vi "log analysis_gps.vi"() -> ()   [LabVIEW 2018] (continued)
INS_RTKFIXED,37.37124990486,126.72244436292,7.9283,22.3000,-0.0470,0.2912,0.0231,-0.374405811,0.178417245,91.756627389,0.4699,0.2842,0.5361,0.1187,0.0913,0.0769,0.1664,0.1677,5.1090,0f000001,0*1daf5624\n\t", "INSPVAXA,USB3,0,47.5,FINESTEERING,2107,281654.050,02000000,471d,15824;INS_ALIGNMENT_COMPLETE,INS_RTKFIXED,37.37124978665,126.72244599017,7.9303,22.3000,-0.0443,0.2911,0.0221,-0.533917833,0.012272263,91.868776619,0.4905,0.2861,0.5500,0.1206,0.0913,0.0777,0.1663,0.1679,5.1083,0f000001,0*b5797700\n\t", "INSPVAXA,USB3,0,50.0,FINESTEERING,2107,281654.550,02000000,471d,15824;INS_ALIGNMENT_COMPLETE,INS_RTKFIXED,37.37124968143,126.72244761542,7.9319,22.3000,-0.0412,0.3115,0.0211,-0.670904223,-0.153080533,91.963880825,0.4905,0.2861,0.5500,0.1206,0.0913,0.0777,0.1663,0.1679,5.1083,0f000001,0*92b26d05\n\t", "INSPVAXA,USB3,0,50.0,FINESTEERING,2107,281655.050,02000000,471d,15824;INS_ALIGNMENT_COMPLETE,INS_RTKFIXED,37.37124956365,126.72244929570,7.9335,22.3000,-0.0287,0.2866,0.0163,-0.633101230,-0.384686660,92.084311938,0.4910,0.2854,0.5548,0.1194,0.0909,0.0776,0.1663,0.1676,5.1075,0f000001,0*34863e77\n\t", "INSPVAXA,USB3,0,45.0,FINESTEERING,2107,281655.550,02000000,471d,15824;INS_ALIGNMENT_COMPLETE,INS_RTKFIXED,37.37124945994,126.72245094764,7.9362,22.3000,-0.0311,0.2897,0.0132,-0.611375277,-0.501090520,92.141784733,0.4910,0.2854,0.5548,0.1194,0.0909,0.0776,0.1663,0.1676,5.1075,0f000001,0*d10d29d1\n\t", "INSPVAXA,USB3,0,45.0,FINESTEERING,2107,281656.050,02000000,471d,15824;INS_ALIGNMENT_COMPLETE,INS_RTKFIXED,37.37124935153,126.72245256975,7.9391,22.3000,-0.0386,0.2989,0.0132,-0.570389168,-0.459677112,92.213933334,0.4880,0.2845,0.5571,0.1182,0.0907,0.0775,0.1662,0.1674,5.1068,0f000001,0*a2bfb50c\n\t", "INSPVAXA,USB3,0,48.5,FINESTEERING,2107,281657.050,02000000,471d,15824;INS_ALIGNMENT_COMPLETE,INS_RTKFIXED,37.37124909812,126.72245582569,7.9380,22.3000,-0.0275,0.2897,0.0035,-0.469663173,-0.125718508,92.311505672,0.4756,0.2829,0.5533,0.1158,0.0905,0.0770,0.1661,0.1672,5.1057,0f000001,0*07acf302\n\t", "INSPVAXA,USB3,0,45.5,FINESTEERING,2107,281657.550,02000000,471d,15824;INS_ALIGNMENT_COMPLETE,INS_RTKFIXED,37.37124898406,126.72245743531,7.9384,22.3000,-0.0303,0.2838,-0.0006,-0.590912103,0.021707043,92.352601821,0.4756,0.2829,0.5533,0.1158,0.0905,0.0770,0.1661,0.1672,5.1057,0f000001,0*08773687\n\t", "INSPVAXA,USB3,0,45.5,FINESTEERING,2107,281658.050,02000000,471d,15824;INS_ALIGNMENT_COMPLETE,INS_RTKFIXED,37.37124887128,126.72245908204,7.9396,22.3000,-0.0216,0.3115,-0.0012,-0.683943291,-0.073848905,92.385513763,0.4705,0.2822,0.5519,0.1155,0.0906,0.0768,0.1661,0.1672,5.1055,0f000001,0*f6b19920\n\t", "INSPVAXA,USB3,0,47.0,FINESTEERING,2107,281658.550,02000000,471d,15824;INS_ALIGNMENT_COMPLETE,INS_RTKFIXED,37.37124877139,126.72246069396,7.9391,22.3000,-0.0206,0.3045,-0.0060,-0.740293612,-0.175653816,92.281973521,0.4705,0.2822,0.5519,0.1155,0.0906,0.0768,0.1661,0.1672,5.1055,0f000001,0*bcff9c67\n\t", "INSPVAXA,USB3,0,47.0,FINESTEERING,2107,281659.050,02000000,471d,15824;INS_ALIGNMENT_COMPLETE,INS_RTKFIXED,37.37124867854,126.72246232189,7.9387,22.3000,-0.0180,0.2907,0.0091,-0.761412694,-0.318240084,92.179006494,0.4753,0.2827,0.5554,0.1164,0.0908,0.0769,0.1661,0.1674,5.1056,0f000001,0*0b8ce59e\n\t", "INSPVAXA,USB3,0,48.0,FINESTEERING,2107,281660.050,02000000,471d,15824;INS_ALIGNMENT_COMPLETE,INS_RTKFIXED,37.37124847032,126.72246556404,7.9397,22.3000,-0.0209,0.3095,-0.0013,-0.677978130,-0.485395170,91.982371596,0.4840,0.2835,0.5609,0.1180,0.0910,0.0772,0.1661,0.1676,5.1059,0f000001,0*3e0b93c3\n\t", "INSPVAXA,USB3,0,49.0,FINESTEERING,2107,281660.550,02000000,471d,15824;INS_ALIGNMENT_COMPLETE,INS_RTKFIXED,37.37124837512,126.72246716631,7.9375,22.3000,-0.0227,0.2996,0.0028,-0.584311559,-0.386112040,91.866898679,0.4840,0.2835,0.5609,0.1180,0.0910,0.0772,0.1661,0.1676,5.1059,0f000001,0*45e2577e\n\t", "INSPVAXA,USB3,0,48.0,FINESTEERING,2107,281661.050,02000000,471d,15824;INS_ALIGNMENT_COMPLETE,INS_RTKFIXED,37.37124829104,126.72246876695,7.9348,22.3000,-0.0195,0.3013,0.0019,-0.605545922,-0.315098575,91.766604977,0.4893,0.2839,0.5649,0.1187,0.0910,0.0774,0.1661,0.1677,5.1061,0f000001,0*33d9cb01\n\t", "INSPVAXA,USB3,0,48.0,FINESTEERING,2107,281662.050,02000000,471d,15824;INS_ALIGNMENT_COMPLETE,INS_RTKFIXED,37.37124811177,126.72247195093,7.9364,22.3000,-0.0115,0.2979,0.0095,-0.572003488,-0.073343292,91.548333593,0.4907,0.2839,0.5665,0.1189,0.0910,0.0775,0.1660,0.1678,5.1065,0f000001,0*28865f95\n\t", "INSPVAXA,USB3,0,49.5,FINESTEERING,2107,281662.550,02000000,471d,15824;INS_ALIGNMENT_COMPLETE,INS_RTKFIXED,37.37124803275,126.72247354020,7.9355,22.3000,-0.0061,0.2831,0.0061,-0.496782272,0.001131440,91.456585867,0.4907,0.2839,0.5665,0.1189,0.0910,0.0775,0.1660,0.1678,5.1065,0f000001,0*47f56ed7\n\t", "INSPVAXA,USB3,0,49.5,FINESTEERING,2107,281663.050,02000000,471d,15824;INS_ALIGNMENT_COMPLETE,INS_RTKFIXED,37.37124795721,126.72247514952,7.9341,22.3000,-0.0032,0.2852,0.0045,-0.477077211,-0.102180757,91.467919397,0.4905,0.2838,0.5669,0.1189,0.0910,0.0775,0.1660,0.1678,5.1072,0f000001,0*7002819d\n\t", "INSPVAXA,USB3,0,50.0,FINESTEERING,2107,281663.550,02000000,471d,15824;INS_ALIGNMENT_COMPLETE,INS_RTKFIXED,37.37124785760,126.72247673495,7.9334,22.3000,-0.0075,0.2892,0.0034,-0.450270802,-0.044143313,91.482502163,0.4905,0.2838,0.5669,0.1189,0.0910,0.0775,0.1660,0.1678,5.1072,0f000001,0*8c44abc3\n\t", "INSPVAXA,USB3,0,49.0,FINESTEERING,2107,281666.550,02000000,471d,15824;INS_ALIGNMENT_COMPLETE,INS_RTKFIXED,37.37124721121,126.72248621902,7.9287,22.3000,-0.0121,0.2777,0.0145,-0.831221770,-0.084392330,92.040205552,0.4814,0.2826,0.5616,0.1182,0.0910,0.0772,0.1659,0.1677,5.1107,0f000001,0*a6e58744\n\t", "INSPVAXA,USB3,0,48.0,FINESTEERING,2107,281667.050,02000000,471d,15824;INS_ALIGNMENT_COMPLETE,INS_RTKFIXED,37.37124708689,126.72248776343,7.9278,22.3000,-0.0198,0.2843,0.0107,-0.784855196,-0.012804695,92.146893043,0.4774,0.2821,0.5586,0.1180,0.0910,0.0771,0.1659,0.1677,5.1116,0f000001,0*9d84455b\n\t", "INSPVAXA,USB3,0,47.0,FINESTEERING,2107,281669.550,02008000,471d,15824;INS_ALIGNMENT_COMPLETE,INS_RTKFIXED,37.37124639381,126.72249565319,7.9242,22.3000,-0.0324,0.2710,-0.0043,-0.728518677,-0.210964710,92.694614055,0.4668,0.2811,0.5506,0.1171,0.0909,0.0768,0.1658,0.1676,5.1128,0f000001,0*35942a2d\n\t", "INSPVAXA,USB3,0,45.0,FINESTEERING,2107,281671.050,02008000,471d,15824;INS_ALIGNMENT_COMPLETE,INS_RTKFIXED,37.37124595365,126.72250039060,7.9180,22.3000,-0.0288,0.2756,-0.0016,-0.760823395,-0.249987892,93.080464082,0.4568,0.2803,0.5426,0.1164,0.0907,0.0766,0.1658,0.1675,5.1134,0f000001,0*bc516aa8\n\t", "INSPVAXA,USB3,0,48.5,FINESTEERING,2107,281688.600,02000000,471d,15824;INS_ALIGNMENT_COMPLETE,INS_RTKFIXED,37.37124079033,126.72255707314,7.9955,22.3000,-0.0400,0.2827,0.0199,-0.588574844,-0.376557071,93.100954007,0.4119,0.2777,0.5056,0.1103,0.0901,0.0751,0.1654,0.1662,5.1286,0f000001,0*54052947\n\t", "INSPVAXA,USB3,0,49.0,FINESTEERING,2107,281692.600,02000000,471d,15824;INS_ALIGNMENT_COMPLETE,INS_RTKFIXED,37.37123920503,126.72256999557,8.0063,22.3000,-0.0578,0.2919,0.0133,-0.505898312,-0.718535643,95.167243727,0.4145,0.2869,0.5143,0.1104,0.0917,0.0756,0.1655,0.1660,5.1296,0f000001,0*c2aa46e2\n\t", "INSPVAXA,USB3,0,47.0,FINESTEERING,2107,281695.100,02000000,471d,15824;INS_ALIGNMENT_COMPLETE,INS_RTKFIXED,37.37123802053,126.72257797318,8.0018,22.3000,-0.0593,0.2857,0.0050,-0.558480992,-0.544515597,95.936874114,0.4188,0.2924,0.5242,0.1107,0.0922,0.0760,0.1653,0.1660,5.1321,0f000001,0*63dd8461\n\t", "INSPVAXA,USB3,0,50.0,FINESTEERING,2107,281696.100,02000000,471d,15824;INS_ALIGNMENT_COMPLETE,INS_RTKFIXED,37.37123750613,126.72258125435,8.0103,22.3000,-0.0675,0.2976,0.0099,-0.630143652,-0.426020851,96.136843189,0.4217,0.2975,0.5312,0.1110,0.0928,0.0763,0.1653,0.1661,5.1333,0f000001,0*1735351b\n\t", "INSPVAXA,USB3,0,48.0,FINESTEERING,2107,281697.100,02000000,471d,15824;INS_ALIGNMENT_COMPLETE,INS_RTKFIXED,37.37123698193,126.72258460282,8.0164,22.3000,-0.0758,0.2921,0.0167,-0.785011326,-0.362402901,96.082518685,0.4231,0.3001,0.5368,0.1110,0.0930,0.0765,0.1653,0.1661,5.1347,0f000001,0*98f592bb\n\t", "INSPVAXA,USB3,0,46.0,FINESTEERING,2107,281698.600,02000000,471d,15824;INS_ALIGNMENT_COMPLETE,INS_RTKFIXED,37.37123629785,126.72258936520,8.0229,22.3000,-0.0531,0.2999,0.0083,-0.429170205,-0.373001381,94.965510664,0.4234,0.2998,0.5394,0.1109,0.0928,0.0765,0.1652,0.1661,5.1363,0f000001,0*f47145af\n\t", "INSPVAXA,USB3,0,47.5,FINESTEERING,2107,281699.100,02000000,471d,15824;INS_ALIGNMENT_COMPLETE,INS_RTKFIXED,37.37123609876,126.72259093053,8.0227,22.3000,-0.0510,0.2765,0.0255,-0.446439369,-0.329194520,94.348853221,0.4489,0.3061,0.5623,0.1153,0.0940,0.0781,0.1653,0.1666,5.1379,0f000001,0*f0667120\n\t", "INSPVAXA,USB3,0,47.5,FINESTEERING,2107,281699.600,02000000,471d,15824;INS_ALIGNMENT_COMPLETE,INS_RTKFIXED,37.37123591668,126.72259250997,8.0220,22.3000,-0.0473,0.2889,0.0139,-0.571559626,-0.354554479,93.825556987,0.4489,0.3061,0.5623,0.1153,0.0940,0.0781,0.1653,0.1666,5.1379,0f000001,0*d2b474b3\n\t", "INSPVAXA,USB3,0,46.5,FINESTEERING,2107,281701.100,02000000,471d,15824;INS_ALIGNMENT_COMPLETE,INS_RTKFIXED,37.37123543674,126.72259726700,8.0121,22.3000,-0.0545,0.2706,0.0002,-0.599049195,-0.261744490,92.339458537,0.4977,0.3169,0.6162,0.1213,0.0953,0.0812,0.1655,0.1673,5.1411,0f000001,0*bffa09db\n\t", "INSPVAXA,USB3,0,46.5,FINESTEERING,2107,281701.600,02000000,471d,15824;INS_ALIGNMENT_COMPLETE,INS_RTKFIXED,37.37123527924,126.72259888049,8.0099,22.3000,-0.0672,0.2799,0.0012,-0.451214464,-0.240273754,91.937158376,0.4977,0.3169,0.6162,0.1213,0.0953,0.0812,0.1655,0.1673,5.1411,0f000001,0*07d7c6e7\n\t", "INSPVAXA,USB3,0,47.5,FINESTEERING,2107,281702.100,02000000,471d,15824;INS_ALIGNMENT_COMPLETE,INS_RTKFIXED,37.37123511620,126.72260050182,8.0076,22.3000,-0.0639,0.2800,0.0071,-0.195522404,-0.345413269,91.687324212,0.5177,0.3188,0.6402,0.1229,0.0952,0.0822,0.1654,0.1675,5.1426,0f000001,0*c86b297b\n\t", "INSPVAXA,USB3,0,47.5,FINESTEERING,2107,281702.600,02000000,471d,15824;INS_ALIGNMENT_COMPLETE,INS_RTKFIXED,37.37123499980,126.72260210723,8.0027,22.3000,-0.0718,0.2769,0.0046,-0.302041493,-0.225202254,91.651416522,0.5177,0.3188,0.6402,0.1229,0.0952,0.0822,0.1654,0.1675,5.1426,0f000001,0*8e66a9f4\n\t", "INSPVAXA,USB3,0,45.0,FINESTEERING,2107,281703.100,02000000,471d,15824;INS_ALIGNMENT_COMPLETE,INS_RTKFIXED,37.37123487466,126.72260370060,7.9985,22.3000,-0.0709,0.2986,0.0115,-0.451708680,-0.253518479,91.680936337,0.5338,0.3195,0.6613,0.1238,0.0951,0.0829,0.1654,0.1676,5.1442,0f000001,0*4cdf9694\n\t", "INSPVAXA,USB3,0,45.0,FINESTEERING,2107,281703.600,02000000,471d,15824;INS_ALIGNMENT_COMPLETE,INS_RTKFIXED,37.37123473881,126.72260531876,7.9953,22.3000,-0.0686,0.2839,0.0069,-0.545599376,-0.327030847,91.675911567,0.5338,0.3195,0.6613,0.1238,0.0951,0.0829,0.1654,0.1676,5.1442,0f000001,0*45031f18\n\t", "INSPVAXA,USB3,0,49.0,FINESTEERING,2107,281704.100,02000000,471d,15824;INS_ALIGNMENT_COMPLETE,INS_RTKFIXED,37.37123458474,126.72260693238,7.9920,22.3000,-0.0673,0.2665,0.0075,-0.425050811,-0.262256492,91.709435128,0.4707,0.3025,0.6068,0.1142,0.0929,0.0788,0.1651,0.1663,5.1457,0f000001,0*e320c835\n\t", "INSPVAXA,USB3,0,49.0,FINESTEERING,2107,281704.600,02000000,471d,15824;INS_ALIGNMENT_COMPLETE,INS_RTKFIXED,37.37123444909,126.72260850935,7.9897,22.3000,-0.0657,0.2780,0.0024,-0.316216564,-0.175738279,91.794051031,0.4707,0.3025,0.6068,0.1142,0.0929,0.0788,0.1651,0.1663,5.1457,0f000001,0*c024accc\n\t", "INSPVAXA,USB3,0,48.5,FINESTEERING,2107,281705.100,02000000,471d,15824;INS_ALIGNMENT_COMPLETE,INS_RTKFIXED,37.37123430154,126.72261008444,7.9873,22.3000,-0.0633,0.2873,0.0036,-0.217542977,-0.113568421,91.893535267,0.4436,0.2955,0.5802,0.1116,0.0926,0.0771,0.1650,0.1661,5.1471,0f000001,0*d440002a\n\t", "INSPVAXA,USB3,0,48.5,FINESTEERING,2107,281705.600,02000000,471d,15824;INS_ALIGNMENT_COMPLETE,INS_RTKFIXED,37.37123415162,126.72261168716,7.9829,22.3000,-0.0703,0.2649,-0.0005,-0.095589755,-0.218915380,92.040147564,0.4436,0.2955,0.5802,0.1116,0.0926,0.0771,0.1650,0.1661,5.1471,0f000001,0*3cc5b35f\n\t", "INSPVAXA,USB3,0,47.0,FINESTEERING,2107,281706.100,02000000,471d,15824;INS_ALIGNMENT_COMPLETE,INS_RTKFIXED,37.37123399063,126.72261326131,7.9791,22.3000,-0.0689,0.2735,0.0004,-0.068217682,-0.338302495,92.198825064,0.4298,0.2917,0.5629,0.1111,0.0926,0.0763,0.1650,0.1662,5.1486,0f000001,0*0d2ba2e9\n\t", "INSPVAXA,USB3,0,47.0,FINESTEERING,2107,281706.600,02000000,471d,15824;INS_ALIGNMENT_COMPLETE,INS_RTKFIXED,37.37123384411,126.72261483687,7.9751,22.3000,-0.0650,0.2968,0.0010,-0.179433418,-0.243858761,92.416884280,0.4298,0.2917,0.5629,0.1111,0.0926,0.0763,0.1650,0.1662,5.1486,0f000001,0*3a14ca69\n\t", "INSPVAXA,USB3,0,46.5,FINESTEERING,2107,281707.100,02000000,471d,15824;INS_ALIGNMENT_COMPLETE,INS_RTKFIXED,37.37123367618,126.72261651459,7.9700,22.3000,-0.0663,0.2892,-0.0095,-0.200364886,-0.287717605,92.565518940,0.4222,0.2895,0.5502,0.1114,0.0926,0.0759,0.1650,0.1662,5.1501,0f000001,0*7d04a348\n\t", "INSPVAXA,USB3,0,46.5,FINESTEERING,2107,281707.600,02000000,471d,15824;INS_ALIGNMENT_COMPLETE,INS_RTKFIXED,37.37123350681,126.72261819185,7.9654,22.3000,-0.0701,0.2829,0.0020,-0.131719254,-0.267188121,92.719108134,0.4222,0.2895,0.5502,0.1114,0.0926,0.0759,0.1650,0.1662,5.1501,0f000001,0*336f6954\n\t", "INSPVAXA,USB3,0,46.5,FINESTEERING,2107,281708.100,02008000,471d,15824;INS_ALIGNMENT_COMPLETE,INS_RTKFIXED,37.37123332387,126.72261975086,7.9614,22.3000,-0.0675,0.2853,0.0025,-0.071583190,-0.126032206,92.932636241,0.4187,0.2881,0.5409,0.1120,0.0926,0.0757,0.1650,0.1662,5.1517,0f000001,0*717a5375\n\t", "INSPVAXA,USB3,0,44.5,FINESTEERING,2107,281708.600,02008000,471d,15824;INS_ALIGNMENT_COMPLETE,INS_RTKFIXED,37.37123313227,126.72262135847,7.9570,22.3000,-0.0735,0.2879,0.0053,-0.006863606,-0.144876749,93.163596493,0.4187,0.2881,0.5409,0.1120,0.0926,0.0757,0.1650,0.1662,5.1517,0f000001,0*5328ad5b\n\t", "INSPVAXA,USB3,0,45.0,FINESTEERING,2107,281709.100,02008000,471d,15824;INS_ALIGNMENT_COMPLETE,INS_RTKFIXED,37.37123292904,126.72262301314,7.9519,22.3000,-0.0859,0.2798,0.0008,-0.080624798,-0.243890207,93.431588866,0.4168,0.2866,0.5328,0.1122,0.0923,0.0756,0.1650,0.1661,5.1533,0f000001,0*5e6ee30b\n\t", "INSPVAXA,USB3,0,45.0,FINESTEERING,2107,281709.600,02008000,471d,15824;INS_ALIGNMENT_COMPLETE,INS_RTKFIXED,37.37123275225,126.72262461471,7.9473,22.3000,-0.0829,0.2713,-0.0040,-0.149358912,-0.219762797,93.778103830,0.4168,0.2866,0.5328,0.1122,0.0923,0.0756,0.1650,0.1661,5.1533,0f000001,0*a588a807\n\t", "INSPVAXA,USB3,0,45.0,FINESTEERING,2107,281710.100,02008000,471d,15824;INS_ALIGNMENT_COMPLETE,INS_RTKFIXED,37.37123256909,126.72262620659,7.9441,22.3000,-0.0800,0.2841,-0.0050,-0.348638579,-0.216651585,94.159342839,0.4165,0.2852,0.5266,0.1124,0.0920,0.0756,0.1649,0.1660,5.1550,0f000001,0*bff3e08f\n\t", "INSPVAXA,USB3,0,49.0,FINESTEERING,2107,281710.600,02008000,471d,15824;INS_ALIGNMENT_COMPLETE,INS_RTKFIXED,37.37123239058,126.72262777304,7.9409,22.3000,-0.0798,0.2944,-0.0023,-0.430611394,-0.234860716,94.547061846,0.4165,0.2852,0.5266,0.1124,0.0920,0.0756,0.1649,0.1660,5.1550,0f000001,0*d6308b3b\n\t", "DUALANTENNAHEADINGA,USB3,0,48.0,FINESTEERING,2107,281711.100,02008000,d426,15824;SOL_COMPUTED,NARROW_FLOAT,-1.000000000,80.289344788,-44.356048584,0.0,300.718536377,180.000000000,\"631T\",19,8,8,8,04,00,20,23*d9de486e\n\t", "INSPVAXA,USB3,0,48.0,FINESTEERING,2107,281711.600,02008000,471d,15824;INS_ALIGNMENT_COMPLETE,INS_RTKFIXED,37.37123199532,126.72263088788,7.9365,22.3000,-0.0807,0.2590,-0.0074,-0.567150366,-0.272813348,95.297147623,0.4157,0.2838,0.5214,0.1122,0.0917,0.0756,0.1649,0.1659,5.1567,0f000001,0*5002614b\n\t", "INSPVAXA,USB3,0,47.5,FINESTEERING,2107,281712.100,02000000,471d,15824;INS_ALIGNMENT_COMPLETE,INS_RTKFIXED,37.37123179004,126.72263242494,7.9368,22.3000,-0.0695,0.2725,-0.0019,-0.650599321,-0.130078123,95.641509239,0.4157,0.2825,0.5179,0.1119,0.0914,0.0757,0.1648,0.1658,5.1583,0f000001,0*44de4a90\n\t", "INSPVAXA,USB3,0,47.5,FINESTEERING,2107,281712.600,02000000,471d,15824;INS_ALIGNMENT_COMPLETE,INS_RTKFIXED,37.37123168411,126.72263304090,7.9346,22.3000,-0.0497,-0.0387,-0.0006,-0.768033993,-0.261504929,95.591408924,0.4157,0.2825,0.5179,0.1119,0.0914,0.0757,0.1648,0.1658,5.1583,0f000001,0*fe46b876\n\t", "INSPVAXA,USB3,0,49.0,FINESTEERING,2107,281713.100,02000000,471d,15824;INS_ALIGNMENT_COMPLETE,INS_RTKFIXED,37.37123162730,126.72263286916,7.9326,22.3000,-0.0467,-0.0089,-0.0011,-0.752184115,-0.247755356,95.681640614,0.4152,0.2811,0.5147,0.1145,0.0912,0.0757,0.1647,0.1656,5.1599,0f000001,0*7f213a14\n\t", "INSPVAXA,USB3,0,49.0,FINESTEERING,2107,281713.600,02000000,471d,15824;INS_ALIGNMENT_COMPLETE,INS_RTKFIXED,37.37123160226,126.72263284212,7.9312,22.3000,-0.0436,-0.0236,-0.0010,-0.754995173,-0.249841362,95.676005261,0.4152,0.2811,0.5147,0.1145,0.0912,0.0757,0.1647,0.1656,5.1599,0f000001,0*48133efc\n\t", "INSPVAXA,USB3,0,49.0,FINESTEERING,2107,281714.100,02000000,471d,15824;INS_ALIGNMENT_COMPLETE,INS_RTKFIXED,37.37123158399,126.72263279406,7.9298,22.3000,-0.0399,-0.0233,-0.0008,-0.760010437,-0.248532428,95.678009350,0.4172,0.2798,0.5120,0.1137,0.0910,0.0756,0.1647,0.1655,5.1584,0f000001,0*814e0d11\n\t", "INSPVAXA,USB3,0,49.0,FINESTEERING,2107,281714.600,02000000,471d,15824;INS_ALIGNMENT_COMPLETE,INS_RTKFIXED,37.37123160799,126.72263276180,7.9284,22.3000,-0.0364,-0.0240,-0.0004,-0.762178806,-0.247643160,95.688059791,0.4172,0.2798,0.5120,0.1137,0.0910,0.0756,0.1647,0.1655,5.1584,0f000001,0*b1bc14cf\n\t", "INSPVAXA,USB3,0,47.5,FINESTEERING,2107,281715.100,02000000,471d,15824;INS_ALIGNMENT_COMPLETE,INS_RTKFIXED,37.37123162975,126.72263271812,7.9272,22.3000,-0.0332,-0.0254,0.0000,-0.763298909,-0.246600758,95.701763966,0.4185,0.2789,0.5100,0.1127,0.0908,0.0756,0.1646,0.1655,5.1528,0f000001,0*0879a17d\n\t", "INSPVAXA,USB3,0,47.5,FINESTEERING,2107,281715.600,02000000,471d,15824;INS_ALIGNMENT_COMPLETE,INS_RTKFIXED,37.37123166929,126.72263269074,7.9254,22.3000,-0.0295,-0.0259,0.0000,-0.763181363,-0.245447561,95.720594560,0.4185,0.2789,0.5100,0.1127,0.0908,0.0756,0.1646,0.1655,5.1528,0f000001,0*8b144437\n\t", "INSPVAXA,USB3,0,47.5,FINESTEERING,2107,281716.100,02000000,471d,15824;INS_ALIGNMENT_COMPLETE,INS_RTKFIXED,37.37123170967,126.72263265292,7.9238,22.3000,-0.0264,-0.0269,-0.0004,-0.764362400,-0.245981262,95.737150322,0.4185,0.2781,0.5083,0.1118,0.0906,0.0755,0.1646,0.1654,5.1445,0f000001,0*f8e3de3b\n\t", "INSPVAXA,USB3,0,48.5,FINESTEERING,2107,281716.600,02000000,471d,15824;INS_ALIGNMENT_COMPLETE,INS_RTKFIXED,37.37123176851,126.72263264285,7.9224,22.3000,-0.0232,-0.0258,0.0004,-0.768584569,-0.246689742,95.757168230,0.4185,0.2781,0.5083,0.1118,0.0906,0.0755,0.1646,0.1654,5.1445,0f000001,0*4a6b11ff\n\t", "INSPVAXA,USB3,0,45.5,FINESTEERING,2107,281717.100,02000000,471d,15824;INS_ALIGNMENT_COMPLETE,INS_RTKFIXED,37.37123177555,126.72263328033,7.9223,22.3000,-0.0576,0.3644,0.0001,-0.832005766,-0.123893266,96.001595857,0.4179,0.2777,0.5069,0.1104,0.0904,0.0755,0.1645,0.1655,5.1359,0f000001,0*38e87445\n\t", "INSPVAXA,USB3,0,45.5,FINESTEERING,2107,281717.600,02000000,471d,15824;INS_ALIGNMENT_COMPLETE,INS_RTKFIXED,37.37123167276,126.72263519972,7.9226,22.3000,-0.0392,0.2146,0.0043,-0.709863436,-0.109995299,96.136679690,0.4179,0.2777,0.5069,0.1104,0.0904,0.0755,0.1645,0.1655,5.1359,0f000001,0*131293dc\n\t", "INSPVAXA,USB3,0,50.0,FINESTEERING,2107,281718.100,02000000,471d,15824;INS_ALIGNMENT_COMPLETE,INS_RTKFIXED,37.37123162511,126.72263648434,7.9220,22.3000,-0.0555,0.3053,-0.0001,-0.719313500,0.029309323,96.356461624,0.4142,0.2776,0.5061,0.1102,0.0903,0.0754,0.1645,0.1655,5.1346,0f000001,0*65443b6e\n\t", "INSPVAXA,USB3,0,50.0,FINESTEERING,2107,281718.600,02000000,471d,15824;INS_ALIGNMENT_COMPLETE,INS_RTKFIXED,37.37123150821,126.72263819990,7.9208,22.3000,-0.0327,0.2368,0.0101,-0.836011591,-0.122473478,96.522319824,0.4142,0.2776,0.5061,0.1102,0.0903,0.0754,0.1645,0.1655,5.1346,0f000001,0*3c509359\n\t", "DUALANTENNAHEADINGA,USB3,0,50.0,FINESTEERING,2107,281719.100,02000000,d426,15824;SOL_COMPUTED,NARROW_FLOAT,-1.000000000,81.686454773,-57.139007568,0.0,241.198776245,172.427688599,\"631T\",19,9,9,9,04,00,20,23*98acc785\n\t", "DUALANTENNAHEADINGA,USB3,0,50.5,FINESTEERING,2107,281719.600,02000000,d426,15824;SOL_COMPUTED,NARROW_FLOAT,-1.000000000,81.772033691,-56.640899658,0.0,242.991180420,178.717849731,\"631T\",19,9,9,9,04,00,20,23*247738d5\n\t", "DUALANTENNAHEADINGA,USB3,0,50.5,FINESTEERING,2107,281720.100,02000000,d426,15824;SOL_COMPUTED,NARROW_FLOAT,-1.000000000,77.492141724,-53.828643799,0.0,241.831039429,180.000000000,\"631T\",18,8,8,8,04,00,20,23*d2631c09\n\t", "INSPVAXA,USB3,0,50.5,FINESTEERING,2107,281720.600,02000000,471d,15824;INS_ALIGNMENT_COMPLETE,INS_RTKFIXED,37.37123091097,126.72264464380,7.9199,22.3000,-0.0398,0.2663,0.0043,-0.781491920,-0.508123165,97.323827994,0.4101,0.2774,0.5047,0.1107,0.0902,0.0753,0.1644,0.1655,5.1368,0f000001,0*f5b81503\n\t", "INSPVAXA,USB3,0,44.0,FINESTEERING,2107,281721.100,02000000,471d,15824;INS_ALIGNMENT_COMPLETE,INS_RTKFIXED,37.37123072966,126.72264623422,7.9185,22.3000,-0.0371,0.2532,0.0002,-0.791450093,-0.646314917,97.497529339,0.4089,0.2773,0.5042,0.1108,0.0902,0.0752,0.1643,0.1654,5.1370,0f000001,0*861aa27e\n\t", "INSPVAXA,USB3,0,44.0,FINESTEERING,2107,281721.600,02000000,471d,15824;INS_ALIGNMENT_COMPLETE,INS_RTKFIXED,37.37123052324,126.72264786246,7.9181,22.3000,-0.0351,0.2700,-0.0076,-0.812155960,-0.930405893,97.703567688,0.4089,0.2773,0.5042,0.1108,0.0902,0.0752,0.1643,0.1654,5.1370,0f000001,0*0ebef3fd\n\t", "DUALANTENNAHEADINGA,USB3,0,44.0,FINESTEERING,2107,281722.100,02000000,d426,15824;SOL_COMPUTED,NARROW_FLOAT,-1.000000000,76.782913208,-57.608184814,0.0,174.641418457,168.358657837,\"631T\",20,9,9,9,04,00,20,23*2ea8cf0f\n\t", "INSPVAXA,USB3,0,47.5,FINESTEERING,2107,281722.600,02000000,471d,15824;INS_ALIGNMENT_COMPLETE,INS_RTKFIXED,37.37123005820,126.72265110077,7.9161,22.3000,-0.0311,0.2570,0.0035,-0.906537656,-1.041249846,98.071868373,0.4085,0.2773,0.5040,0.1115,0.0902,0.0751,0.1642,0.1654,5.1358,0f000001,0*21f04e37\n\t", "INSPVAXA,USB3,0,46.5,FINESTEERING,2107,281723.100,02000000,471d,15824;INS_ALIGNMENT_COMPLETE,INS_RTKFIXED,37.37122980766,126.72265265100,7.9163,22.3000,-0.0386,0.2513,-0.0019,-0.889198276,-0.870105161,98.274091102,0.4388,0.2808,0.5181,0.1159,0.0909,0.0762,0.1643,0.1660,5.1342,0f000001,0*96582036\n\t", "INSPVAXA,USB3,0,46.5,FINESTEERING,2107,281723.600,02000000,471d,15824;INS_ALIGNMENT_COMPLETE,INS_RTKFIXED,37.37122953819,126.72265422237,7.9162,22.3000,-0.0387,0.2553,0.0003,-0.677469280,-0.596133835,98.468377537,0.4388,0.2808,0.5181,0.1159,0.0909,0.0762,0.1643,0.1660,5.1342,0f000001,0*0344c34f\n\t", "INSPVAXA,USB3,0,50.0,FINESTEERING,2107,281724.100,02000000,471d,15824;INS_ALIGNMENT_COMPLETE,INS_RTKFIXED,37.37122926408,126.72265582006,7.9155,22.3000,-0.0392,0.2664,0.0052,-0.552231420,-0.356374368,98.612981561,0.4681,0.2838,0.5347,0.1192,0.0914,0.0772,0.1643,0.1664,5.1316,0f000001,0*5ab7c900\n\t", "DUALANTENNAHEADINGA,USB3,0,50.0,FINESTEERING,2107,281724.600,02000000,d426,15824;SOL_COMPUTED,NARROW_FLOAT,-1.000000000,73.725341797,-44.577819824,0.0,216.156219482,180.000000000,\"631T\",18,6,6,6,04,00,20,03*eb9ec7a2\n\t", "DUALANTENNAHEADINGA,USB3,0,48.0,FINESTEERING,2107,281725.100,02000000,d426,15824;SOL_COMPUTED,NARROW_FLOAT,-1.000000000,77.386466980,-38.596252441,0.0,347.977569580,180.000000000,\"631T\",17,7,7,6,04,00,20,33*9a5ac747\n\t", "DUALANTENNAHEADINGA,USB3,0,48.0,FINESTEERING,2107,281725.600,02000000,d426,15824;SOL_COMPUTED,NARROW_FLOAT,-1.000000000,74.226867676,-38.265563965,0.0,314.182830811,180.000000000,\"631T\",17,7,7,6,04,00,20,23*45cb672d\n\t", "DUALANTENNAHEADINGA,USB3,0,48.0,FINESTEERING,2107,281726.100,02000000,d426,15824;SOL_COMPUTED,NARROW_FLOAT,-1.000000000,204.498168945,55.872886658,0.0,207.629287720,89.946952820,\"631T\",18,5,5,5,04,00,20,03*b03bb7fc\n\t", "DUALANTENNAHEADINGA,USB3,0,49.5,FINESTEERING,2107,281726.600,02000000,d426,15824;SOL_COMPUTED,NARROW_FLOAT,-1.000000000,205.496963501,57.094558716,0.0,186.765380859,78.783508301,\"631T\",22,5,5,5,04,00,20,03*8aea4973\n\t", "INSPVAXA,USB3,0,40.0,FINESTEERING,2107,281727.100,02000000,471d,15824;INS_ALIGNMENT_COMPLETE,INS_RTKFIXED,37.37122812563,126.72266113643,7.9335,22.3000,-0.0046,-0.0366,0.0030,-0.538484803,-0.008426097,98.999278684,0.4214,0.2780,0.5150,0.1122,0.0902,0.0752,0.1639,0.1653,5.1250,0f000001,0*ffbd65c8\n\t", "DUALANTENNAHEADINGA,USB3,0,40.0,FINESTEERING,2107,281727.600,02000000,d426,15824;SOL_COMPUTED,NARROW_FLOAT,-1.000000000,200.788482666,48.749797821,0.0,300.075164795,180.000000000,\"631T\",21,7,7,7,04,00,20,33*2f30a934\n\t", "DUALANTENNAHEADINGA,USB3,0,40.0,FINESTEERING,2107,281728.100,02000000,d426,15824;SOL_COMPUTED,NARROW_FLOAT,-1.000000000,68.682434082,-18.649810791,0.0,214.877609253,180.000000000,\"631T\",24,9,9,7,04,00,20,33*477f08c5\n\t", "INSPVAXA,USB3,0,47.5,FINESTEERING,2107,281728.600,02000000,471d,15824;INS_ALIGNMENT_COMPLETE,INS_RTKFIXED,37.37122802316,126.72266112148,7.9338,22.3000,-0.0028,-0.0273,0.0028,-0.537660493,-0.013430681,99.001211572,0.4185,0.2775,0.5119,0.1116,0.0903,0.0750,0.1638,0.1653,5.1258,0f000001,0*537c1130\n\t", "DUALANTENNAHEADINGA,USB3,0,40.0,FINESTEERING,2107,281729.100,02000000,d426,15824;SOL_COMPUTED,NARROW_FLOAT,-1.000000000,109.638298035,-31.887359619,0.0,360.000000000,180.000000000,\"631T\",23,10,10,8,04,00,20,33*61c9d85b\n\t", "DUALANTENNAHEADINGA,USB3,0,40.0,FINESTEERING,2107,281729.600,02000000,d426,15824;SOL_COMPUTED,NARROW_FLOAT,-1.000000000,110.155059814,-31.497802734,0.0,360.000000000,180.000000000,\"631T\",22,10,10,8,04,00,20,23*86070080\n\t", "DUALANTENNAHEADINGA,USB3,0,40.0,FINESTEERING,2107,281730.100,02000000,d426,15824;SOL_COMPUTED,NARROW_FLOAT,-1.000000000,72.987403870,-66.832275391,0.0,145.125228882,72.779129028,\"631T\",22,9,9,9,04,00,20,33*22d7f0e2\n\t", "DUALANTENNAHEADINGA,USB3,0,44.5,FINESTEERING,2107,281730.600,02000000,d426,15824;SOL_COMPUTED,NARROW_FLOAT,-1.000000000,73.134811401,-67.340759277,0.0,145.030975342,70.451110840,\"631T\",24,8,8,8,04,00,20,23*a3bb5097\n\t", "DUALANTENNAHEADINGA,USB3,0,44.5,FINESTEERING,2107,281731.100,02000000,d426,15824;SOL_COMPUTED,NARROW_FLOAT,-1.000000000,67.550712585,-53.724426270,0.0,93.597503662,81.789405823,\"631T\",24,11,11,8,04,00,20,33*f2cdb2de\n\t", "DUALANTENNAHEADINGA,USB3,0,46.0,FINESTEERING,2107,281731.600,02000000,d426,15824;SOL_COMPUTED,NARROW_FLOAT,-1.000000000,67.703987122,-53.717529297,0.0,93.903839111,81.812553406,\"631T\",25,11,11,8,04,00,20,33*84af30bc\n\t", "DUALANTENNAHEADINGA,USB3,0,46.0,FINESTEERING,2107,281732.100,02000000,d426,15824;SOL_COMPUTED,NARROW_FLOAT,-1.000000000,70.648727417,-51.742156982,0.0,100.178024292,90.939315796,\"631T\",24,9,9,8,04,00,20,33*a1cde6a3\n\t", "DUALANTENNAHEADINGA,USB3,0,48.5,FINESTEERING,2107,281732.600,02000000,d426,15824;SOL_COMPUTED,NARROW_FLOAT,-1.000000000,71.467155457,-52.314849854,0.0,103.026306152,90.018371582,\"631T\",24,9,9,7,04,00,20,33*b7826648\n\t", "DUALANTENNAHEADINGA,USB3,0,46.5,FINESTEERING,2107,281733.100,02000000,d426,15824;SOL_COMPUTED,NARROW_FLOAT,-1.000000000,126.205139160,18.349567413,0.0,360.000000000,180.000000000,\"631T\",24,8,8,7,04,00,20,33*2d8a4dce\n\t", "DUALANTENNAHEADINGA,USB3,0,46.5,FINESTEERING,2107,281733.600,02000000,d426,15824;SOL_COMPUTED,NARROW_FLOAT,-1.000000000,128.837829590,37.580234528,0.0,360.000000000,180.000000000,\"631T\",23,8,8,7,04,00,20,33*aad36c56\n\t", "DUALANTENNAHEADINGA,USB3,0,46.5,FINESTEERING,2107,281734.100,02000000,d426,15824;SOL_COMPUTED,L1_FLOAT,-1.000000000,224.733520508,68.118484497,0.0,40.168888092,35.261268616,\"631T\",23,9,9,8,04,00,20,32*6f92941a\n\t", "DUALANTENNAHEADINGA,USB3,0,49.0,FINESTEERING,2107,281734.600,02000000,d426,15824;SOL_COMPUTED,L1_FLOAT,-1.000000000,224.765914917,68.098785400,0.0,40.323402405,35.416801453,\"631T\",24,9,9,8,04,00,20,32*7247d44b\n\t", "DUALANTENNAHEADINGA,USB3,0,49.0,FINESTEERING,2107,281735.100,02000000,d426,15824;SOL_COMPUTED,NARROW_FLOAT,-1.000000000,130.053359985,14.075355530,0.0,360.000000000,180.000000000,\"631T\",24,8,8,7,04,00,20,33*3c5b7a30\n\t", "DUALANTENNAHEADINGA,USB3,0,49.5,FINESTEERING,2107,281735.600,02000000,d426,15824;SOL_COMPUTED,NARROW_FLOAT,-1.000000000,129.132507324,11.961747169,0.0,360.000000000,180.000000000,\"631T\",23,8,8,7,04,00,20,33*3d51ce5b\n\t", "DUALANTENNAHEADINGA,USB3,0,49.0,FINESTEERING,2107,281736.100,02000000,d426,15824;SOL_COMPUTED,NARROW_FLOAT,-1.000000000,66.459640503,-9.324951172,0.0,167.365310669,180.000000000,\"631T\",23,11,11,7,04,00,20,33*cd3bb081\n\t", "DUALANTENNAHEADINGA,USB3,0,49.0,FINESTEERING,2107,281736.600,02000000,d426,15824;SOL_COMPUTED,NARROW_FLOAT,-1.000000000,65.953575134,-8.853302002,0.0,164.536880493,180.000000000,\"631T\",23,11,11,7,04,00,20,33*7a71c18e\n\t", "DUALANTENNAHEADINGA,USB3,0,48.0,FINESTEERING,2107,281737.100,02000000,d426,15824;SOL_COMPUTED,NARROW_FLOAT,-1.000000000,177.908920288,86.914611816,0.0,360.000000000,93.604774475,\"631T\",23,9,9,9,04,00,20,32*986b758d\n\t", "DUALANTENNAHEADINGA,USB3,0,48.0,FINESTEERING,2107,281737.600,02000000,d426,15824;SOL_COMPUTED,NARROW_FLOAT,-1.000000000,175.774688721,87.167266846,0.0,360.000000000,89.855789185,\"631T\",24,8,8,8,04,00,20,32*9d4057da\n\t", "DUALANTENNAHEADINGA,USB3,0,48.0,FINESTEERING,2107,281738.100,02000000,d426,15824;SOL_COMPUTED,NARROW_FLOAT,-1.000000000,69.591072083,21.682659149,0.0,219.854476929,180.000000000,\"631T\",24,11,11,8,04,00,20,33*690f967f\n\t", "DUALANTENNAHEADINGA,USB3,0,44.0,FINESTEERING,2107,281739.100,02000000,d426,15824;SOL_COMPUTED,NARROW_FLOAT,-1.000000000,64.034339905,-17.544586182,0.0,156.327194214,180.000000000,\"631T\",24,11,11,10,04,00,20,23*2589d380\n\t", "DUALANTENNAHEADINGA,USB3,0,44.0,FINESTEERING,2107,281740.100,02000000,d426,15824;SOL_COMPUTED,NARROW_FLOAT,-1.000000000,74.082733154,-10.455871582,0.0,242.974914551,180.000000000,\"631T\",25,10,10,8,04,00,20,33*2f825e02\n\t", "DUALANTENNAHEADINGA,USB3,0,47.0,FINESTEERING,2107,281741.100,02000000,d426,15824;SOL_COMPUTED,NARROW_FLOAT,-1.000000000,85.015144348,31.514696121,0.0,312.612518311,180.000000000,\"631T\",25,11,11,10,04,00,20,33*b44ad5e5\n\t", "DUALANTENNAHEADINGA,USB3,0,47.0,FINESTEERING,2107,281741.600,02000000,d426,15824;SOL_COMPUTED,NARROW_FLOAT,-1.000000000,83.672279358,32.063629150,0.0,308.060882568,180.000000000,\"631T\",26,11,11,9,04,00,20,33*4b707776\n\t", "DUALANTENNAHEADINGA,USB3,0,48.0,FINESTEERING,2107,281742.600,02000000,d426,15824;SOL_COMPUTED,NARROW_FLOAT,-1.000000000,70.145378113,-51.275817871,0.0,227.918136597,180.000000000,\"631T\",25,9,9,9,04,00,20,33*d9969f72\n\t", "DUALANTENNAHEADINGA,USB3,0,44.0,FINESTEERING,2107,281743.600,02000000,d426,15824;SOL_COMPUTED,NARROW_FLOAT,-1.000000000,80.124595642,-25.270904541,0.0,308.231628418,180.000000000,\"631T\",24,11,11,8,04,00,20,33*e319a4f8\n\t", "DUALANTENNAHEADINGA,USB3,0,44.0,FINESTEERING,2107,281744.100,02000000,d426,15824;SOL_COMPUTED,NARROW_FLOAT,-1.000000000,88.668289185,-42.090301514,0.0,218.729476929,180.000000000,\"631T\",27,12,12,8,04,00,20,33*7e036603\n\t", "DUALANTENNAHEADINGA,USB3,0,43.0,FINESTEERING,2107,281745.100,02000000,d426,15824;SOL_COMPUTED,L1_FLOAT,-1.000000000,76.229156494,-52.514221191,0.0,343.746551514,180.000000000,\"631T\",24,8,8,8,04,00,20,22*58ffa7a9\n\t", "INSPVAXA,USB3,0,43.0,FINESTEERING,2107,281745.650,02000000,471d,15824;INS_ALIGNMENT_COMPLETE,INS_RTKFIXED,37.37122376712,126.72269430723,7.9696,22.3000,0.0009,-0.0216,0.0069,-0.151476991,-0.103231506,94.688643057,0.4242,0.2996,0.5710,0.1152,0.0935,0.0773,0.1637,0.1653,5.0964,0f000001,0*7621de5b\n\t", "DUALANTENNAHEADINGA,USB3,0,43.0,FINESTEERING,2107,281746.100,02000000,d426,15824;SOL_COMPUTED,NARROW_FLOAT,-1.000000000,80.487289429,-0.437042236,0.0,264.792785645,180.000000000,\"631T\",23,11,11,9,04,00,20,33*333581cd\n\t", "INSPVAXA,USB3,0,48.5,FINESTEERING,2107,281746.650,02000000,471d,15824;INS_ALIGNMENT_COMPLETE,INS_RTKFIXED,37.37122367686,126.72269432693,7.9700,22.3000,-0.0006,-0.0203,0.0085,-0.151258490,-0.103499239,94.673524903,0.4235,0.2995,0.5674,0.1146,0.0934,0.0772,0.1636,0.1652,5.0926,0f000001,0*5a88747a\n\t", "DUALANTENNAHEADINGA,USB3,0,47.0,FINESTEERING,2107,281747.100,02000000,d426,15824;SOL_COMPUTED,NARROW_FLOAT,-1.000000000,79.948493958,-1.148895264,0.0,261.968414307,180.000000000,\"631T\",25,11,11,8,04,00,20,33*bccd161e\n\t", "INSPVAXA,USB3,0,47.0,FINESTEERING,2107,281747.650,02000000,471d,15824;INS_ALIGNMENT_COMPLETE,INS_RTKFIXED,37.37122361083,126.72269434828,7.9719,22.3000,-0.0025,-0.0192,0.0107,-0.148677227,-0.104675299,94.662876541,0.4231,0.2994,0.5645,0.1138,0.0934,0.0773,0.1636,0.1650,5.0876,0f000001,0*63e2391f\n\t", "DUALANTENNAHEADINGA,USB3,0,47.0,FINESTEERING,2107,281748.100,02000000,d426,15824;SOL_COMPUTED,NARROW_FLOAT,-1.000000000,79.773033142,-38.986785889,0.0,161.515747070,180.000000000,\"631T\",26,14,14,9,04,00,20,23*3f0231ce\n\t", "INSPVAXA,USB3,0,47.0,FINESTEERING,2107,281748.650,02000000,471d,15824;INS_ALIGNMENT_COMPLETE,INS_RTKFIXED,37.37122355418,126.72269437706,7.9761,22.3000,-0.0041,-0.0183,0.0125,-0.147280099,-0.105053583,94.655580641,0.4227,0.2992,0.5623,0.1131,0.0933,0.0773,0.1635,0.1648,5.0828,0f000001,0*cff9a17d\n\t", "DUALANTENNAHEADINGA,USB3,0,47.0,FINESTEERING,2107,281749.100,02000000,d426,15824;SOL_COMPUTED,NARROW_FLOAT,-1.000000000,78.765502930,-35.557800293,0.0,142.700469971,180.000000000,\"631T\",25,9,9,9,04,00,20,23*972183bf\n\t", "INSPVAXA,USB3,0,47.0,FINESTEERING,2107,281749.650,02000000,471d,15824;INS_ALIGNMENT_COMPLETE,INS_RTKFIXED,37.37122336848,126.72269668314,7.9846,22.3000,-0.0207,0.2294,0.0088,-0.275967163,-0.168126378,94.547495368,0.4219,0.2990,0.5605,0.1123,0.0932,0.0774,0.1635,0.1647,5.0793,0f000001,0*31f4ca89\n\t", "DUALANTENNAHEADINGA,USB3,0,47.0,FINESTEERING,2107,281750.100,02000000,d426,15824;SOL_COMPUTED,NARROW_FLOAT,-1.000000000,73.333755493,-58.579284668,0.0,229.934936523,180.000000000,\"631T\",23,9,9,9,04,00,20,23*088e0644\n\t", "INSPVAXA,USB3,0,49.0,FINESTEERING,2107,281750.650,02000000,471d,15824;INS_ALIGNMENT_COMPLETE,INS_RTKFIXED,37.37122306940,126.72269984285,7.9912,22.3000,-0.0257,0.2957,0.0077,-0.057724950,-0.163350878,94.045578333,0.4218,0.2990,0.5600,0.1154,0.0932,0.0775,0.1634,0.1646,5.0783,0f000001,0*27ab5aaa\n\t", "INSPVAXA,USB3,0,44.0,FINESTEERING,2107,281751.150,02000000,471d,15824;INS_ALIGNMENT_COMPLETE,INS_RTKFIXED,37.37122292112,126.72270145835,7.9931,22.3000,-0.0258,0.2880,0.0101,-0.111536572,-0.252430525,93.709532324,0.4176,0.2990,0.5591,0.1145,0.0931,0.0775,0.1634,0.1645,5.0797,0f000001,0*615311ce\n\t", "DUALANTENNAHEADINGA,USB3,0,44.0,FINESTEERING,2107,281751.600,02000000,d426,15824;SOL_COMPUTED,NARROW_FLOAT,-1.000000000,110.156936646,-9.428588867,0.0,360.000000000,180.000000000,\"631T\",23,8,8,8,04,00,20,33*43819e80\n\t", "INSPVAXA,USB3,0,48.0,FINESTEERING,2107,281752.150,02000000,471d,15824;INS_ALIGNMENT_COMPLETE,INS_RTKFIXED,37.37122265407,126.72270470547,8.0012,22.3000,-0.0341,0.2842,0.0130,-0.222146581,-0.505161594,92.535665637,0.4393,0.3011,0.5700,0.1180,0.0937,0.0785,0.1633,0.1649,5.0792,0f000001,0*a665f62f\n\t", "INSPVAXA,USB3,0,47.0,FINESTEERING,2107,281753.150,02000000,471d,15824;INS_ALIGNMENT_COMPLETE,INS_RTKFIXED,37.37122240940,126.72270799161,8.0105,22.3000,-0.0212,0.2738,0.0106,-0.057702421,-0.540115409,91.679699760,0.4576,0.3026,0.5817,0.1199,0.0939,0.0793,0.1633,0.1651,5.0754,0f000001,0*cdf942d8\n\t", "INSPVAXA,USB3,0,49.5,FINESTEERING,2107,281754.150,02000000,471d,15824;INS_ALIGNMENT_COMPLETE,INS_RTKFIXED,37.37122220677,126.72271122628,8.0166,22.3000,-0.0162,0.2741,0.0138,-0.137895898,-0.319145604,91.130640627,0.4709,0.3035,0.5925,0.1202,0.0941,0.0798,0.1633,0.1651,5.0690,0f000001,0*5011df6e\n\t", "INSPVAXA,USB3,0,47.5,FINESTEERING,2107,281755.150,02000000,471d,15824;INS_ALIGNMENT_COMPLETE,INS_RTKFIXED,37.37122201064,126.72271448049,8.0208,22.3000,-0.0166,0.2736,0.0165,-0.348957996,-0.224906485,91.007651183,0.4789,0.3039,0.6014,0.1198,0.0941,0.0802,0.1633,0.1650,5.0614,0f000001,0*7ee29d08\n\t", "INSPVAXA,USB3,0,47.5,FINESTEERING,2107,281755.650,02000000,471d,15824;INS_ALIGNMENT_COMPLETE,INS_RTKFIXED,37.37122187648,126.72271611793,8.0227,22.3000,-0.0203,0.2843,0.0276,-0.262004326,-0.178495771,91.033181464,0.4789,0.3039,0.6014,0.1198,0.0941,0.0802,0.1633,0.1650,5.0614,0f000001,0*fdcbd20c\n\t", "INSPVAXA,USB3,0,48.5,FINESTEERING,2107,281756.150,02000000,471d,15824;INS_ALIGNMENT_COMPLETE,INS_RTKFIXED,37.37122173906,126.72271771096,8.0239,22.3000,-0.0196,0.2676,0.0157,-0.262264917,-0.227266763,91.141814343,0.4824,0.3038,0.6077,0.1190,0.0941,0.0803,0.1632,0.1648,5.0544,0f000001,0*6ba67688\n\t", "INSPVAXA,USB3,0,48.5,FINESTEERING,2107,281756.650,02000000,471d,15824;INS_ALIGNMENT_COMPLETE,INS_RTKFIXED,37.37122160314,126.72271932823,8.0233,22.3000,-0.0269,0.2666,0.0159,-0.432031669,-0.241379053,91.270317292,0.4824,0.3038,0.6077,0.1190,0.0941,0.0803,0.1632,0.1648,5.0544,0f000001,0*d136edd6\n\t", "INSPVAXA,USB3,0,46.0,FINESTEERING,2107,281757.150,02000000,471d,15824;INS_ALIGNMENT_COMPLETE,INS_RTKFIXED,37.37122146617,126.72272086261,8.0239,22.3000,-0.0238,0.2505,0.0126,-0.539342745,-0.282143344,91.361763043,0.4827,0.3037,0.6118,0.1183,0.0941,0.0803,0.1632,0.1647,5.0490,0f000001,0*c068de04\n\t", "INSPVAXA,USB3,0,45.0,FINESTEERING,2107,281758.150,02008000,471d,15824;INS_ALIGNMENT_COMPLETE,INS_RTKFIXED,37.37122126174,126.72272085859,8.0222,22.3000,-0.0253,0.0078,0.0138,-0.584106594,-0.271120528,91.359411557,0.4805,0.3034,0.6136,0.1183,0.0941,0.0802,0.1631,0.1646,5.0450,0f000001,0*5d21a2ee\n\t", "INSPVAXA,USB3,0,48.0,FINESTEERING,2107,281759.150,02008000,471d,15824;INS_ALIGNMENT_COMPLETE,INS_RTKFIXED,37.37122108214,126.72272080985,8.0198,22.3000,-0.0260,-0.0094,0.0141,-0.568558330,-0.274735846,91.351120657,0.4775,0.3029,0.6135,0.1183,0.0941,0.0800,0.1631,0.1645,5.0455,0f000001,0*eb7ab8d8\n\t", "INSPVAXA,USB3,0,48.0,FINESTEERING,2107,281759.650,02008000,471d,15824;INS_ALIGNMENT_COMPLETE,INS_RTKFIXED,37.37122103098,126.72272079622,8.0204,22.3000,-0.0250,-0.0120,0.0146,-0.568680900,-0.276246354,91.350467693,0.4775,0.3029,0.6135,0.1183,0.0941,0.0800,0.1631,0.1645,5.0455,0f000001,0*f26d72a9\n\t", "INSPVAXA,USB3,0,49.0,FINESTEERING,2107,281760.650,02008000,471d,15824;INS_ALIGNMENT_COMPLETE,INS_RTKFIXED,37.37122097057,126.72272075488,8.0199,22.3000,-0.0212,-0.0129,0.0148,-0.569283262,-0.275679751,91.347037233,0.5005,0.3048,0.6288,0.1214,0.0945,0.0808,0.1631,0.1649,5.0468,0f000001,0*fe34bbca\n\t", "INSPVAXA,USB3,0,45.0,FINESTEERING,2107,281761.150,02008000,471d,15824;INS_ALIGNMENT_COMPLETE,INS_RTKFIXED,37.37122095791,126.72272073406,8.0193,22.3000,-0.0189,-0.0135,0.0143,-0.568902262,-0.276160283,91.348963154,0.5200,0.3063,0.6436,0.1235,0.0947,0.0816,0.1630,0.1651,5.0472,0f000001,0*0a850e4d\n\t", "INSPVAXA,USB3,0,45.0,FINESTEERING,2107,281761.650,02008000,471d,15824;INS_ALIGNMENT_COMPLETE,INS_RTKFIXED,37.37122095627,126.72272072968,8.0191,22.3000,-0.0178,0.0000,0.0152,-0.570572969,-0.261989481,91.327306860,0.5200,0.3063,0.6436,0.1235,0.0947,0.0816,0.1630,0.1651,5.0472,0f000001,0*036a1cc5\n\t", "INSPVAXA,USB3,0,48.5,FINESTEERING,2107,281762.150,02008000,471d,15824;INS_ALIGNMENT_COMPLETE,INS_RTKFIXED,37.37122093950,126.72272215279,8.0206,22.3000,-0.0488,0.3741,0.0233,-0.705475481,-0.265236590,91.294421038,0.5354,0.3074,0.6573,0.1254,0.0948,0.0822,0.1629,0.1651,5.0466,0f000001,0*f62868a6\n\t", "INSPVAXA,USB3,0,48.5,FINESTEERING,2107,281762.650,02008000,471d,15824;INS_ALIGNMENT_COMPLETE,INS_RTKFIXED,37.37122090398,126.72272383903,8.0212,22.3000,-0.0171,0.2083,0.0195,-0.539847805,-0.389561252,91.382608507,0.5354,0.3074,0.6573,0.1254,0.0948,0.0822,0.1629,0.1651,5.0466,0f000001,0*ee4bab04\n\t", "INSPVAXA,USB3,0,45.5,FINESTEERING,2107,281763.150,02000000,471d,15824;INS_ALIGNMENT_COMPLETE,INS_RTKFIXED,37.37122088109,126.72272535886,8.0227,22.3000,-0.0346,0.3404,0.0283,-0.600883432,-0.278437530,91.419884915,0.5438,0.3081,0.6694,0.1254,0.0948,0.0826,0.1629,0.1651,5.0479,0f000001,0*0f3b6f6b\n\t", "INSPVAXA,USB3,0,45.5,FINESTEERING,2107,281763.650,02000000,471d,15824;INS_ALIGNMENT_COMPLETE,INS_RTKFIXED,37.37122084767,126.72272697455,8.0246,22.3000,-0.0147,0.2375,0.0201,-0.753001308,-0.365484631,91.444706948,0.5438
